vi "Amplitude_compare.vi"() -> ()   [LabVIEW 2016]
panel:
  in  "stop":bool
  out "x-y":dbl[](array[numeric])
  out "Waveform Graph":dbl[][](graph)
  in  "length":i32
  in  "subarray":dbl[](array[numeric])=array[9600 elements]
  in  "Input":dbl[](array[numeric])=array[5119 elements]
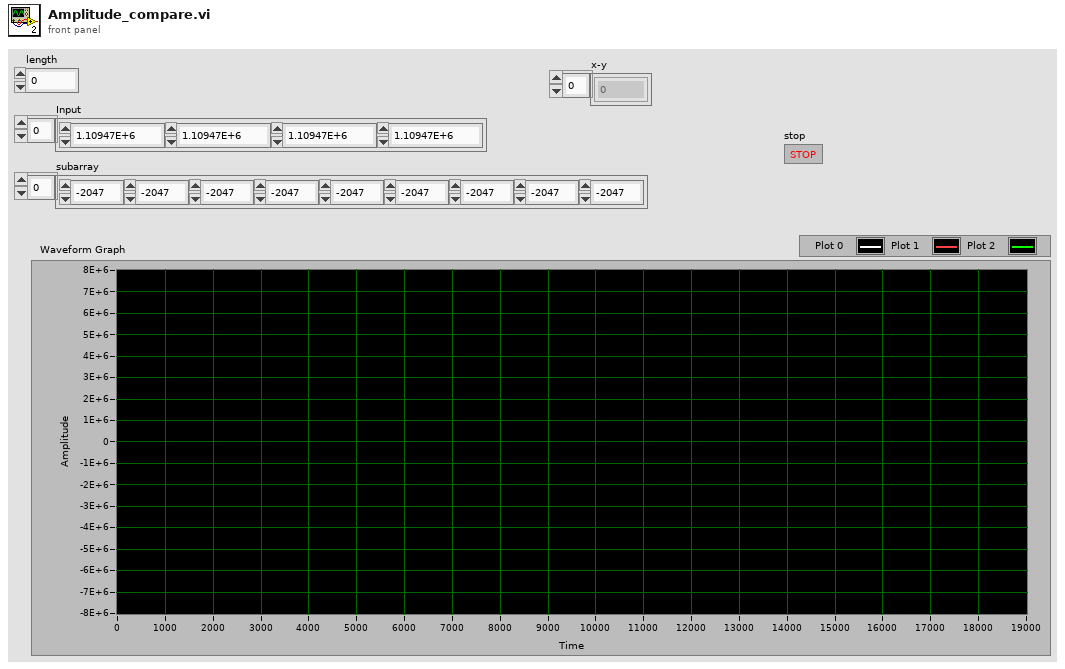
[diagram p1: front panel]
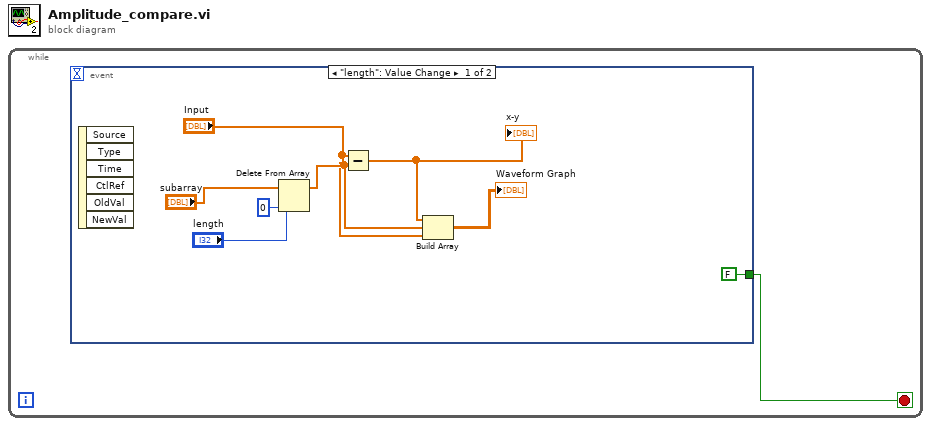
[diagram p0: block diagram]
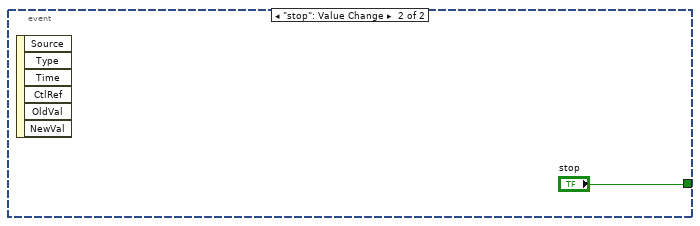
[diagram p2: hidden frame]
diagram:
  n1 = while {
    stop <- w1 stop-if-true
    n2 = event shown="[0] \"length\": Value Change" {
      selector: _ -> [_ _]
      dyn-events: _ -> [_ _]
      timeout: _ -> [_ _]
      tunnel: [FALSE ("stop") "stop"] -> w1
      event "length": Value Change {
        n3 = event-data() -> ()  [unwired: 1 in, 6 out]
        n4 = Delete From Array(array="subarray", length="length", index=0) -> (array with subset deleted=w4:dbl[])  [unwired: 1 out]
        n5 = Subtract(x="Input", y=w4) -> (x-y=w5:dbl[])
        "x-y" <- w5
        n6 = Build Array(w5, w4, "Input") -> (→"Waveform Graph":dbl[][])
      }
      event "stop": Value Change {
        n7 = event-data() -> ()  [unwired: 1 in, 6 out]
      }
    }
  }
